vi "Yaw Crossover.vi"(9 "Target Adjusted Yaw":dbl, 10 "Yaw in":dbl, 11 "Adjustment":dbl) -> (3 "Numeric out":dbl)   [LabVIEW 2018]
panel:
  out "Adjusted Yaw":dbl
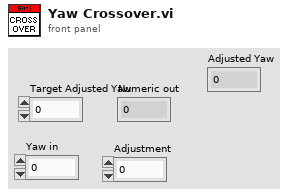
[diagram p1: front panel]
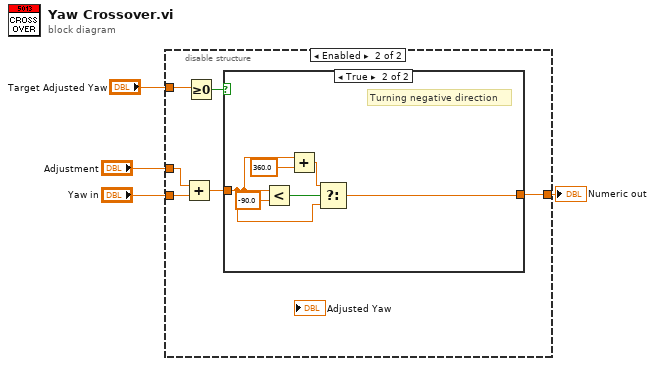
[diagram p0: block diagram]
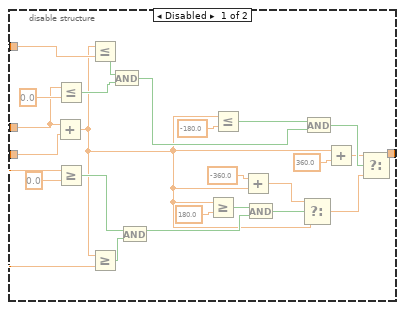
[diagram p2: hidden frame]
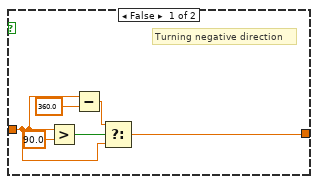
[diagram p3: hidden frame]
diagram:
  n1 = disable-structure shown="Enabled" {
    disable-tunnel: [w17 w29] -> w4
    disable-tunnel: "Yaw in" -> [w16 w32]
    disable-tunnel: "Adjustment" -> [w7 w31]
    disable-tunnel: "Target Adjusted Yaw" -> [w6 w33]
    frame Disabled {
      n2 = Add(x=w7, y=w16) -> (x+y=w5:dbl)
      n3 = Less Or Equal?(x=w7, y=0.0 ("Y-Axis")) -> (x <= y?=w12:bool)
      n4 = Greater Or Equal?(x=w7, y=0.0 ("Y-Axis")) -> (x >= y?=w13:bool)
      n5 = Less Or Equal?(x=w5, y=w6) -> (x <= y?=w10:bool)
      n6 = Greater Or Equal?(x=w5, y=w6) -> (x >= y?=w8:bool)
      n7 = And(x=w10, y=w12) -> (x .and. y?=w11:bool)
      n8 = And(x=w13, y=w8) -> (x .and. y?=w9:bool)
      n9 = Greater Or Equal?(x=w5, y=180.0) -> (x >= y?=w22:bool)
      n10 = Less Or Equal?(x=w5, y=-180.0) -> (x <= y?=w27:bool)
      n11 = Add(x=-360.0, y=w5) -> (x+y=w19:dbl)
      n12 = And(x=w22, y=w9) -> (x .and. y?=w21:bool)
      n13 = Select(t=w19, s=w21, f=w5) -> (s? t:f=w18:dbl)
      n14 = And(x=w27, y=w11) -> (x .and. y?=w26:bool)
      n15 = Add(x=w5, y=360.0) -> (x+y=w24:dbl)
      n16 = Select(t=w24, s=w26, f=w18) -> (s? t:f=w17:dbl)
    }
    frame Enabled {
      n17 = Add(x=w31, y=w32) -> (x+y=w30:dbl)
      n18 = Greater Or Equal To 0?(x=w33) -> (x >= 0?=w34:bool)
      n19 = case shown="True" w34 {
        tunnel: w30 -> [w36 w42]
        tunnel: [w35 w41] -> w29
        frame False {
          # "Turning negative direction"
          n20 = Greater?(x=w36, y=90.0) -> (0:w37:bool)
          n21 = Subtract(x=w36, y=360.0) -> (x-y=w38:dbl)
          n22 = Select(t=w38, s=w37, f=w36) -> (s? t:f=w35:dbl)
        }
        frame True {
          # "Turning negative direction"
          n23 = Less?(x=w42, y=-90.0) -> (x < y?=w43:bool)
          n24 = Add(x=w42, y=360.0) -> (x+y=w44:dbl)
          n25 = Select(t=w44, s=w43, f=w42) -> (s? t:f=w41:dbl)
        }
      }
    }
  }
  "Numeric out" <- w4
